vi "CaseStructure Test 1.vi"   [LabVIEW 2014]
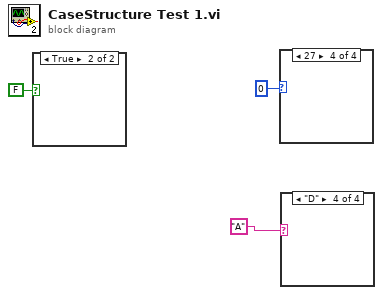
[diagram p0: block diagram]
diagram:
  n1 = case shown="True" FALSE {
    frame False {
    }
    frame True {
    }
  }
  n2 = case shown="27" 0 {
    frame 0, Default {
    }
    frame 1 {
    }
    frame 42 {
    }
    frame 27 {
    }
  }
  n3 = case shown="\"D\"" "A" {
    frame "A", Default {
    }
    frame "B" {
    }
    frame "C" {
    }
    frame "D" {
    }
  }
